vi "Script Constant VI.vi"(7 "Custom Argument Window":refnum<vi>, 8 "error in":errorcluster, 11 "VI Reference":refnum<vi>) -> (0 "error out":errorcluster, 3 "VI reference":refnum<vi>)   [LabVIEW 2020, in "ConstantErrorsMaker.lvlib"]
uses:
  <vilib>/Utility/traverseref.llb/TRef TravTarget.ctl
  <vilib>/Utility/miscctls.llb/LVPositionTypeDef.ctl
  ConstantErrorsMaker.lvlib
  <vilib>/Utility/traverseref.llb/VI Scripting - Traverse.lvlib
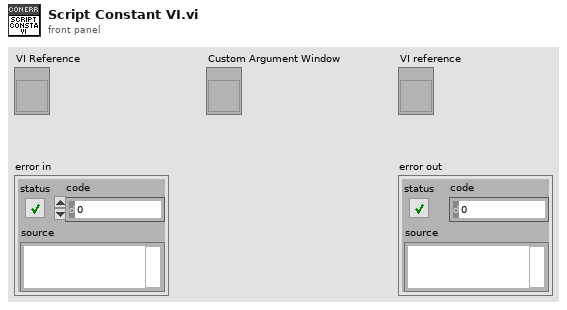
[diagram p1: front panel]
types:
  T1 = typedef "TRef TravTarget.ctl" = enum16{"FP", "BD", "Other"}
  T2 = typedef "LVPositionTypeDef.ctl" = cluster{"Left":i32, "Top":i32}
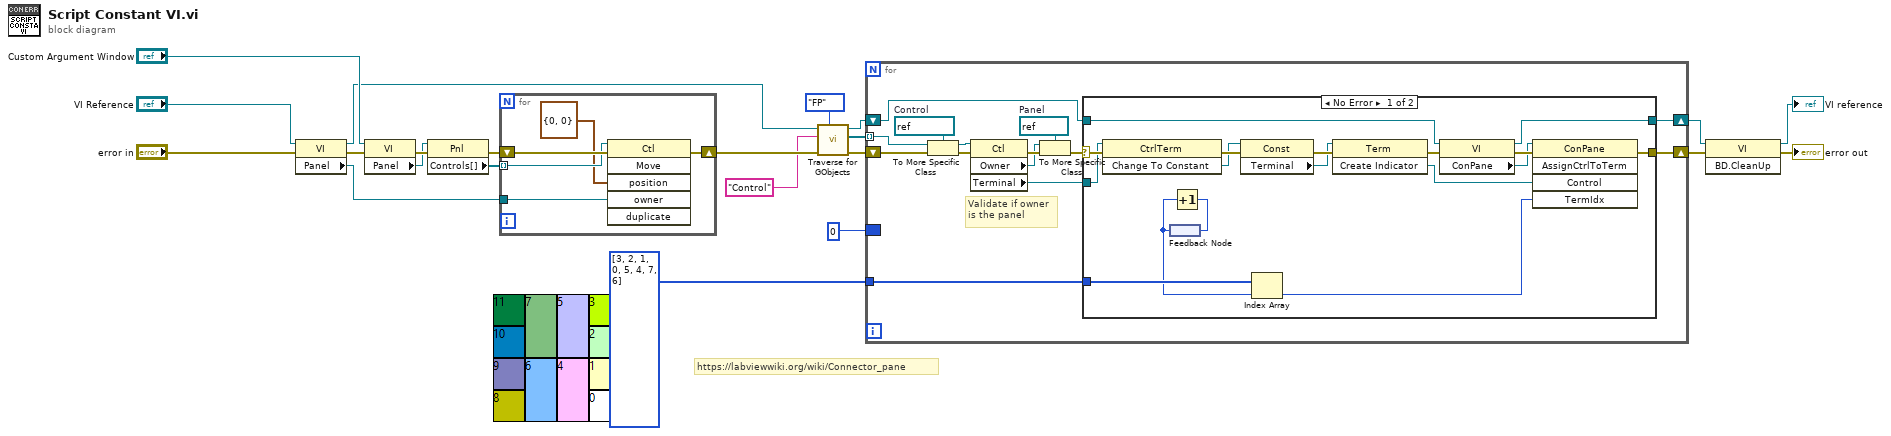
[diagram p0: block diagram]
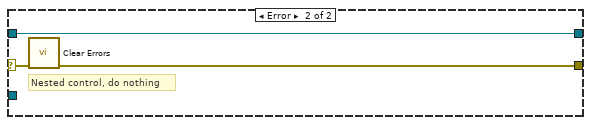
[diagram p2: hidden frame]
diagram:
  # "https://labviewwiki.org/wiki/Connector_pane"
  n1 = property class="VI"(reference="VI Reference", error in="error in") -> (reference out=w9:refnum<vi>, error out=w19:errorcluster, "Panel"=w11:refnum<vi>)
  n2 = property class="VI"(reference="Custom Argument Window", error in=w19) -> (error out=w21:errorcluster, "Panel"=w13:refnum<vi>)  [unwired: 1 out]
  n3 = property class="Pnl"(reference=w13, error in=w21) -> (error out=w20:errorcluster, "Controls[]"=w12:refnum<vi>[])  [unwired: 1 out]
  n4 = for {
    tunnel: w12 -> [w25] mode=indexing
    shift-right: [w26] -> w17
    shift-left: w20 -> [w27]
    tunnel: w11 -> [w24]
    n5 = invoke class="Ctl" method="Move"(reference=w25, error in=w27, "position"=T2 {"Left"=0, "Top"=0}, "owner"=w24) -> (error out=w26:errorcluster)  [unwired: 2 in, 5 out]
  }
  n6 = call <vilib>:"Traverse for GObjects.vi"("Traverse Target"=TRef_TravTarget."FP", "error in (no error)"=w17, "Class Name"="Control", "VI Refnum"=w9) -> ("error out"=w16:errorcluster, "References"=w2:refnum<vi>[], "dup VI Refnum"=w3:refnum<vi>)  [unwired: 4 in, 1 out]
  n7 = for {
    tunnel: i32[] [3, 2, 1, 0, 5, 4, 7, 6] -> [w36]
    tunnel: w2 -> [w31] mode=indexing
    shift-right: [w41] -> w18
    shift-left: w16 -> [w40]
    shift-right: [w35] -> w6
    shift-left: w3 -> [w34]
    border: 0 -> [_]
    w30 = refnum<vi> refnum  # Panel
    w32 = refnum<vi> refnum  # Control
    # "Validate if owner\nis the panel"
    n8 = To More Specific Class(target class=w32, reference=w31, error in=w40) -> (specific class reference=w33:refnum<vi>, error out=w39:errorcluster)
    n9 = property class="Ctl"(reference=w33, error in=w39) -> (error out=w38:errorcluster, "Owner"=w28:refnum<vi>, "Terminal"=w29:refnum<vi>)  [unwired: 1 out]
    n10 = To More Specific Class(target class=w30, reference=w28, error in=w38) -> (error out=w37:errorcluster)  [unwired: 1 out]
    n11 = case shown="No Error" w37 {
      selector: w37 -> [w55 w61]
      tunnel: [w57 w60] -> w41
      tunnel: w36 -> [w46 _]
      tunnel: [w50 w59] -> w35
      tunnel: w34 -> [w49 w59]
      tunnel: w29 -> [w43 _]
      frame No Error {
        n12 = invoke class="CtrlTerm" method="Change To Constant"(reference=w43, error in=w55) -> (error out=w54:errorcluster, "Change To Constant"=w48:refnum<vi>)  [unwired: 1 in, 1 out]
        n13 = feedback #1() -> (w42:i32)
        n14 = Increment(x=w42) -> (x+1=w44:i32)
        n15 = feedback-in #1(w44) -> ()
        n16 = property class="Const"(reference=w48, error in=w54) -> (error out=w53:errorcluster, "Terminal"=w47:refnum<vi>)  [unwired: 1 out]
        n17 = Index Array(array=w46, index=w42) -> (element=w45:i32)
        n18 = invoke class="Term" method="Create Indicator"(reference=w47, error in=w53) -> (error out=w56:errorcluster, "Create Indicator"=w51:refnum<vi>)  [unwired: 1 in, 1 out]
        n19 = property class="VI"(reference=w49, error in=w56) -> (reference out=w50:refnum<vi>, error out=w58:errorcluster, "ConPane"=w52:refnum<vi>)
        n20 = invoke class="ConPane" method="AssignCtrlToTerm"(reference=w52, error in=w58, "Control"=w51, "TermIdx"=w45) -> (error out=w57:errorcluster)  [unwired: 1 in, 4 out]
      }
      frame Error {
        # "Nested control, do nothing"
        n21 = call <vilib>:"Clear Errors.vi"("error in (no error)"=w61) -> ("error out"=w60:errorcluster)  [unwired: 5 in, 1 out]
      }
    }
  }
  n22 = invoke class="VI" method="BD.CleanUp"(reference=w6, error in=w18) -> (reference out=→"VI reference":refnum<vi>, error out=→"error out":errorcluster)  [unwired: 1 in, 1 out]
